vi "create_date_array.vi"() -> (3 "Date Array":string[](array[string]))   [LabVIEW 2016]
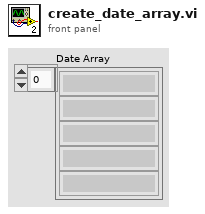
[diagram p1: front panel]
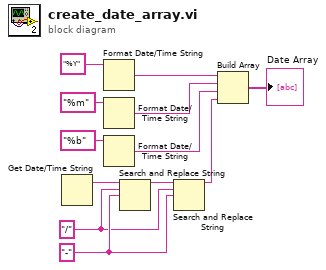
[diagram p0: block diagram]
diagram:
  w7 = "-"
  w6 = "/"
  n1 = Get Date/Time String() -> (date string=w4:string)  [unwired: 3 in, 1 out]
  n2 = Format Date/Time String(time format string (%c)="%Y") -> (date/time string=w8:string)  [unwired: 2 in]
  n3 = Format Date/Time String(time format string (%c)="%m") -> (date/time string=w9:string)  [unwired: 2 in]
  n4 = Format Date/Time String(time format string (%c)="%b") -> (date/time string=w10:string)  [unwired: 2 in]
  n5 = Search and Replace String(input string=w4, search string=w6, replace string=w7) -> (result string=w5:string)  [unwired: 5 in, 3 out]
  n6 = Search and Replace String(input string=w5, search string=w6, replace string=w7) -> (result string=w11:string)  [unwired: 5 in, 3 out]
  n7 = Build Array(w8, w9, w10, w11) -> (→"Date Array":string[])
